vi "Pixi cam.vi"   [LabVIEW 2017]
uses:
  <vilib>/Rock Robotics/SystemInterfaces/spilib/spi_bus.ctl
  PixyCamSPI.vi
types:
  T1 = typedef "spi_bus.ctl" = enum16{"SPI On-Board, CS0", "SPI On-Board, CS1", "SPI On-Board, CS2", "SPI On-Board, CS3", "SPI MXP", "Invalid"}
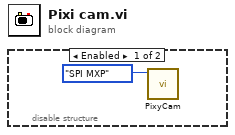
[diagram p0: block diagram]
diagram:
  n1 = disable-structure shown="Enabled" {
    frame Enabled {
      n2 = call-poly "PixyCam.vi"("SPI Bus"=spi_bus."SPI MXP") -> ()  [unwired: 11 in]
    }
    frame Disabled {
    }
  }
